vi "Get KFM names from PGserver.vi"(6 "conninfo":T2={"host"="localhost", "port"="5432", "client_encoding"="WIN1251", "dbname"="data", "user"="postgres", "password"=""}, 8 "error in (no error)":errorcluster, 9 "KFMParamColumns":string[](array[string])=["MVIName", "fcode_full"], 10 "KFMParamTable":string="kfm_3", 11 "KFMParameters":string[](array[string])) -> (0 "error out":errorcluster, 3 "MVINames":string[](array[string]))   [LabVIEW 2021]
uses:
  PostgreSQL/PostgreSQL2LabVIEW/ctl/Coninfo.ctl
  PostgreSQL/PostgreSQL2LabVIEW/libpqlv/src/PQfinish.vi
  PostgreSQL/PostgreSQL2LabVIEW/libpqlv/src/PQconnectdb.vi
  PostgreSQL/PostgreSQL2LabVIEW/libpqlv/src/PQerrorMessage.vi
  PostgreSQL/PostgreSQL2LabVIEW/libpqlv/src/PQstatus.vi
  <vilib>/dlg_ctls.llb/Space Constant.vi
  PostgreSQL/PostgreSQL2LabVIEW/libpqUtility/libpqutility.lvlib
  PostgreSQL/PostgreSQL.lvlib
panel:
  out "progress 3":i32
  out "PQStatus":T1(ring)
  # "MVIName"
  # "fcode_full"
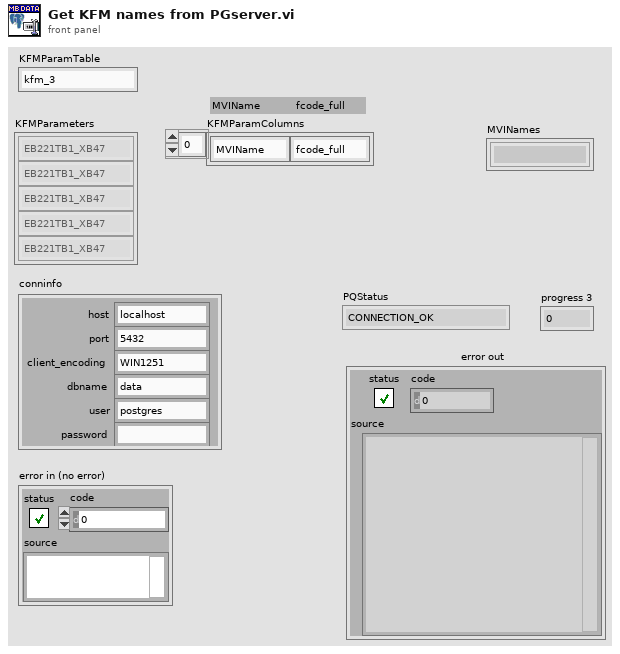
[diagram p1: front panel]
types:
  T1 = enum32{"CONNECTION_OK", "CONNECTION_BAD", "CONNECTION_STARTED", "CONNECTION_MADE", "CONNECTION_AWAITING_RESPONSE", "CONNECTION_AUTH_OK", "CONNECTION_SETENV", "CONNECTION_SSL_STARTUP", "CONNECTION_NEEDED"}
  T2 = typedef "libpqutility.lvlib/Coninfo.ctl" = cluster{"host":string, "port":string, "client_encoding":string, "dbname":string, "user":string, "password":string}
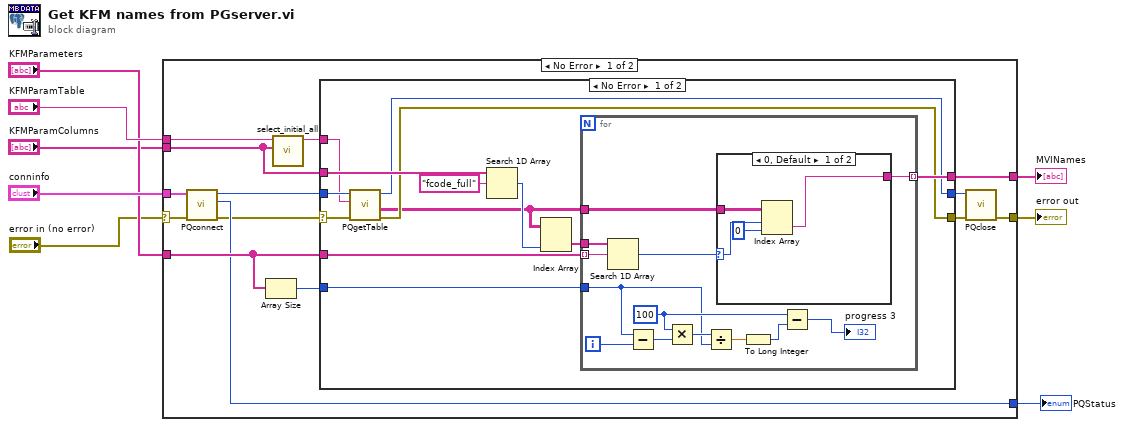
[diagram p0: block diagram]
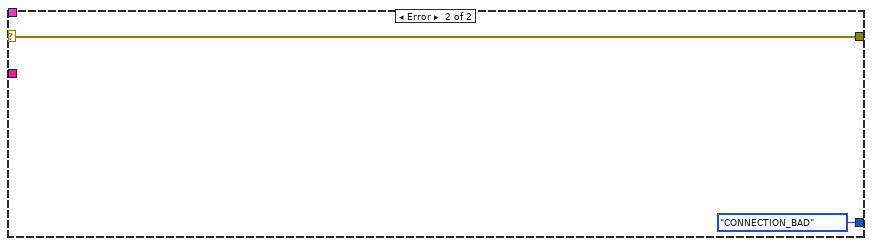
[diagram p4: hidden frame]
diagram:
  n1 = case shown="No Error" "error in (no error)" {
    selector: "error in (no error)" -> [w17 w56]
    tunnel: [w22 w56] -> w8
    tunnel: "KFMParamColumns" -> [w21 _]
    tunnel: "conninfo" -> [w20 _]
    tunnel: "KFMParamTable" -> [w19 _]
    tunnel: "KFMParameters" -> [w18 _]
    tunnel: [w16 T1."CONNECTION_BAD" ("PQStatus")] -> w3
    tunnel: [w15 _] -> w1
    frame No Error {
      n2 = call "PQconnect.vi"("error in (no error)"=w17, "conninfo"=w20) -> ("error out"=w11:errorcluster, "PQStatus"=w16:T1, "conn"=w12:u64)  [unwired: 7 in]
      n3 = Array Size(array=w18) -> (size(s)=w14:i32)
      n4 = call "select_initial_all.vi"("Column table"=w21, "table"=w19) -> ("parameters"=w13:string)  [unwired: 8 in, 1 out]
      n5 = case shown="No Error" w11 {
        selector: w11 -> [w23 w54]
        tunnel: w18 -> [w34 _]
        tunnel: w14 -> [w35 _]
        tunnel: w12 -> [w27 w53]
        tunnel: w13 -> [w26 _]
        tunnel: [w28 w54] -> w10
        tunnel: [w25 w53] -> w9
        tunnel: [w33 _] -> w15
        tunnel: w21 -> [w29 _]
        frame No Error {
          n6 = call "PQgetTable.vi"("error in"=w23, "query"=w26, "conn"=w27) -> ("error out"=w28:errorcluster, "Data"=w24:string[][], "conn_out"=w25:u64)  [unwired: 4 in, 2 out]
          n7 = Search 1D Array(1D array=w29, element="fcode_full" ("table")) -> (index of element=w31:i32)  [unwired: 1 in]
          n8 = Index Array(array=w24, index (col)=w31) -> (element=w30:string[])  [unwired: 1 in]
          n9 = for {
            tunnel: w35 -> [w42]
            tunnel: w34 -> [w37] mode=indexing
            tunnel: [w40] -> w33 mode=indexing
            tunnel: w24 -> [w39]
            tunnel: w30 -> [w38]
            i -> [w43]
            w47 = 100 ("y")
            n10 = Search 1D Array(1D array=w38, element=w37) -> (index of element=w36:i32)  [unwired: 1 in]
            n11 = Subtract(x=w42, y=w43) -> (x-y=w46:i32)
            n12 = Multiply(x=w47, y=w46) -> (x*y=w48:i32)
            n13 = Divide(x=w48, y=w42) -> (x/y=w45:dbl)
            n14 = case shown="0, Default" w36 {
              selector: w36 -> [w51 _]
              tunnel: [w49 _] -> w40
              tunnel: w39 -> [w52 _]
              frame 0, Default {
                n15 = Index Array(array=w52, index (row)=w51, index (col)=0 ("disabled index (col)")) -> (element=w49:string)
              }
              frame -1 {
              }
            }
            n16 = To Long Integer(number=w45) -> (32bit integer=w44:i32)
            n17 = Subtract(x=w47, y=w44) -> (x-y=→"progress 3":i32)
          }
        }
        frame Error {
        }
      }
      n18 = call "PQclose.vi"("error in (no error)"=w10, "conn"=w9) -> ("error out"=w22:errorcluster)  [unwired: 9 in]
    }
    frame Error {
    }
  }
  "error out" <- w8
  "PQStatus" <- w3
  "MVINames" <- w1
